vi "Change Configuration.vi"(1 "input cluster":T1 {"MaxLambdaCurrent [A]" format="%.3f"; "LambdaRates [A/min]" format="%.2f"; "MaxNormalCurrent [A]" format="%.3f"; "StabilitySetting [%]" format="%.2f"; "FieldCurrentRatio [T/A]" format="%.6f"; "SwitchWaitTime [s]" format="%.2f"; "SwitchHtrCurrent [mA]" format="%.2f"; "TrainRates [A/min]" format="%.2f"; "NormalRates [A/min]" format="%.2f"; "Breakpts [A]" format="%.3f"}, 3 "VISA session":refnum<visa-resource-name>="GPIB0::22::INSTR") -> (0 "Output cluster":T1 {"MaxLambdaCurrent [A]" format="%.2f"; "LambdaRates [A/min]" format="%.2f"; "MaxNormalCurrent [A]" format="%.2f"; "StabilitySetting [%]" format="%.2f"; "FieldCurrentRatio [T/A]" format="%.2f"; "SwitchWaitTime [s]" format="%.2f"; "SwitchHtrCurrent [mA]" format="%.2f"; "TrainRates [A/min]" format="%.2f"; "NormalRates [A/min]" format="%.2f"; "Breakpts [A]" format="%.2f"})   [LabVIEW 2019]
panel:
  in  "OK Button":bool
  # "Change parameters below then hit OK\nchanges will be written to the PS and \nthe configuration file"
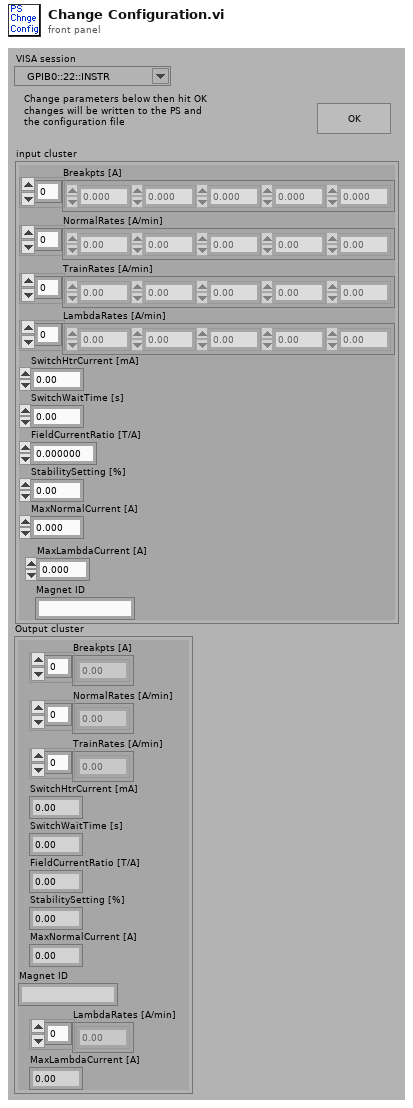
[diagram p1: front panel]
types:
  T1 = cluster{"Breakpts [A]":dbl[], "NormalRates [A/min]":dbl[], "TrainRates [A/min]":dbl[], "SwitchHtrCurrent [mA]":dbl, "SwitchWaitTime [s]":dbl, "FieldCurrentRatio [T/A]":dbl, "StabilitySetting [%]":dbl, "MaxNormalCurrent [A]":dbl, "Magnet ID":string, "LambdaRates [A/min]":dbl[], "MaxLambdaCurrent [A]":dbl}
  T2 = enum16{"Normal", "Train", "Lambda", "Train & Lambda"}
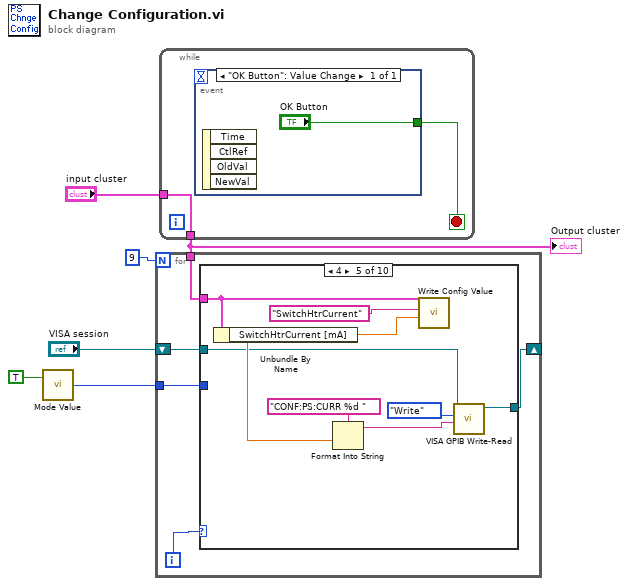
[diagram p0: block diagram]
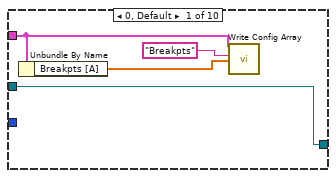
[diagram p2: hidden frame]
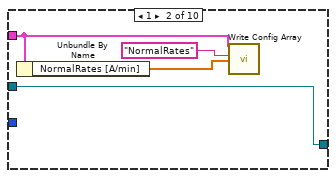
[diagram p3: hidden frame]
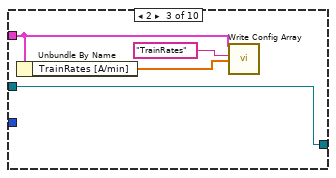
[diagram p4: hidden frame]
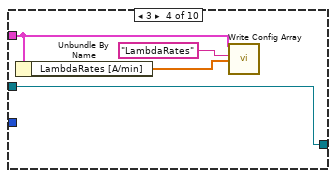
[diagram p5: hidden frame]
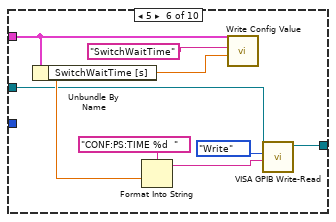
[diagram p6: hidden frame]
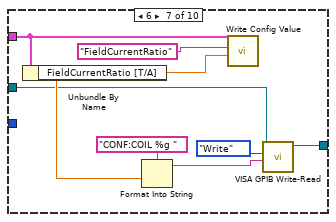
[diagram p7: hidden frame]
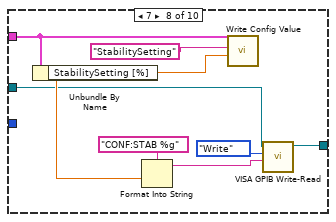
[diagram p8: hidden frame]
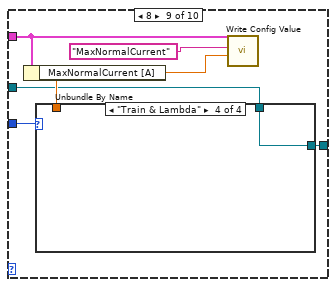
[diagram p9: hidden frame]
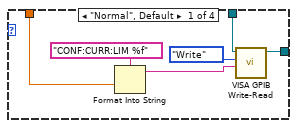
[diagram p10: hidden frame]
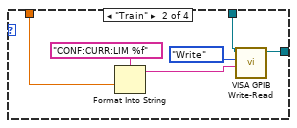
[diagram p11: hidden frame]
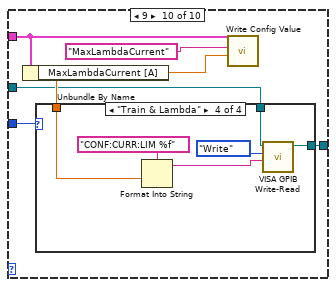
[diagram p13: hidden frame]
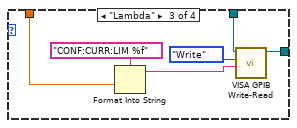
[diagram p16: hidden frame]
diagram:
  n1 = call "Mode Value.vi"("Read/Write this vi"=TRUE) -> ("Mode Out"=w2:T2)  [unwired: 1 in]
  n2 = while {
    tunnel: "input cluster" -> [w7]
    tunnel: [w7] -> w4
    stop <- w8 stop-if-true
    n3 = event shown="[0] \"OK Button\": Value Change" {
      selector: _ -> [_]
      dyn-events: _ -> [_]
      timeout: _ -> [_]
      tunnel: ["OK Button"] -> w8
      event "OK Button": Value Change {
        n4 = event-data() -> ()  [unwired: 1 in, 4 out]
      }
    }
  }
  "Output cluster" <- w4
  n5 = for {
    N: 9 -> [_]
    tunnel: w4 -> [w13]
    tunnel: w2 -> [w12]
    shift-right: [w10] -> _
    shift-left: "VISA session" -> [w11]
    i -> [w14]
    n6 = case shown="4" w14 {
      tunnel: w13 -> [w18 w22 w26 w30 w38 w46 w54 w62 w68 w88]
      tunnel: w12 -> [_ _ _ _ _ _ _ _ w65 w85]
      tunnel: w11 -> [w15 w19 w23 w27 w32 w40 w48 w56 w64 w84]
      tunnel: [w15 w19 w23 w27 w31 w39 w47 w55 w63 w83] -> w10
      frame 0, Default {
        n7 = Unbundle By Name(w18) -> ("Breakpts [A]"=w16:dbl[])
        n8 = call "Write Config Array.vi"("array"=w16, "Key"="Breakpts", "input cluster"=w18) -> ()  [unwired: 1 in, 2 out]
      }
      frame 1 {
        n9 = Unbundle By Name(w22) -> ("NormalRates [A/min]"=w20:dbl[])
        n10 = call "Write Config Array.vi"("array"=w20, "Key"="NormalRates", "input cluster"=w22) -> ()  [unwired: 1 in, 2 out]
      }
      frame 2 {
        n11 = Unbundle By Name(w26) -> ("TrainRates [A/min]"=w24:dbl[])
        n12 = call "Write Config Array.vi"("array"=w24, "Key"="TrainRates", "input cluster"=w26) -> ()  [unwired: 1 in, 2 out]
      }
      frame 3 {
        n13 = Unbundle By Name(w30) -> ("LambdaRates [A/min]"=w28:dbl[])
        n14 = call "Write Config Array.vi"("array"=w28, "Key"="LambdaRates", "input cluster"=w30) -> ()  [unwired: 1 in, 2 out]
      }
      frame 4 {
        n15 = Unbundle By Name(w38) -> ("SwitchHtrCurrent [mA]"=w36:dbl)
        n16 = Format Into String(format string="CONF:PS:CURR %d " ("Command String"), w36) -> (resulting string=w34:string)  [unwired: 2 in, 1 out]
        n17 = call "Write Config Value.vi"("Value"=w36, "Key"="SwitchHtrCurrent", "input cluster"=w38) -> ()  [unwired: 1 in, 2 out]
        n18 = call "VISA GPIB Write-Read.vi"("Command"=w34, "Action"=enum16{"Write", "Read", "Write & Read"}."Write", "VISA resource name"=w32) -> ("dup VISA Session"=w31:refnum<visa-resource-name>)  [unwired: 5 in, 3 out]
      }
      frame 5 {
        n19 = Unbundle By Name(w46) -> ("SwitchWaitTime [s]"=w44:dbl)
        n20 = Format Into String(format string="CONF:PS:TIME %d  " ("Command String"), w44) -> (resulting string=w43:string)  [unwired: 2 in, 1 out]
        n21 = call "Write Config Value.vi"("Value"=w44, "Key"="SwitchWaitTime", "input cluster"=w46) -> ()  [unwired: 1 in, 2 out]
        n22 = call "VISA GPIB Write-Read.vi"("Command"=w43, "Action"=enum16{"Write", "Read", "Write & Read"}."Write", "VISA resource name"=w40) -> ("dup VISA Session"=w39:refnum<visa-resource-name>)  [unwired: 5 in, 3 out]
      }
      frame 6 {
        n23 = Unbundle By Name(w54) -> ("FieldCurrentRatio [T/A]"=w52:dbl)
        n24 = Format Into String(format string="CONF:COIL %g " ("Command String"), w52) -> (resulting string=w50:string)  [unwired: 2 in, 1 out]
        n25 = call "Write Config Value.vi"("Value"=w52, "Key"="FieldCurrentRatio", "input cluster"=w54) -> ()  [unwired: 1 in, 2 out]
        n26 = call "VISA GPIB Write-Read.vi"("Command"=w50, "Action"=enum16{"Write", "Read", "Write & Read"}."Write", "VISA resource name"=w48) -> ("dup VISA Session"=w47:refnum<visa-resource-name>)  [unwired: 5 in, 3 out]
      }
      frame 7 {
        n27 = Unbundle By Name(w62) -> ("StabilitySetting [%]"=w60:dbl)
        n28 = Format Into String(format string="CONF:STAB %g" ("Command String"), w60) -> (resulting string=w58:string)  [unwired: 2 in, 1 out]
        n29 = call "Write Config Value.vi"("Value"=w60, "Key"="StabilitySetting", "input cluster"=w62) -> ()  [unwired: 1 in, 2 out]
        n30 = call "VISA GPIB Write-Read.vi"("Command"=w58, "Action"=enum16{"Write", "Read", "Write & Read"}."Write", "VISA resource name"=w56) -> ("dup VISA Session"=w55:refnum<visa-resource-name>)  [unwired: 5 in, 3 out]
      }
      frame 8 {
        n31 = Unbundle By Name(w68) -> ("MaxNormalCurrent [A]"=w66:dbl)
        n32 = case shown="\"Train & Lambda\"" w65 {
          tunnel: w66 -> [w74 w80 _ _]
          tunnel: w64 -> [w70 w76 w81 w82]
          tunnel: [w69 w75 w81 w82] -> w63
          frame "Normal", Default {
            n33 = Format Into String(format string="CONF:CURR:LIM %f" ("Command String"), w74) -> (resulting string=w72:string)  [unwired: 2 in, 1 out]
            n34 = call "VISA GPIB Write-Read.vi"("Command"=w72, "Action"=enum16{"Write", "Read", "Write & Read"}."Write", "VISA resource name"=w70) -> ("dup VISA Session"=w69:refnum<visa-resource-name>)  [unwired: 5 in, 3 out]
          }
          frame "Train" {
            n35 = Format Into String(format string="CONF:CURR:LIM %f" ("Command String"), w80) -> (resulting string=w78:string)  [unwired: 2 in, 1 out]
            n36 = call "VISA GPIB Write-Read.vi"("Command"=w78, "Action"=enum16{"Write", "Read", "Write & Read"}."Write", "VISA resource name"=w76) -> ("dup VISA Session"=w75:refnum<visa-resource-name>)  [unwired: 5 in, 3 out]
          }
          frame "Lambda" {
          }
          frame "Train & Lambda" {
          }
        }
        n37 = call "Write Config Value.vi"("Value"=w66, "Key"="MaxNormalCurrent", "input cluster"=w68) -> ()  [unwired: 1 in, 2 out]
      }
      frame 9 {
        n38 = Unbundle By Name(w88) -> ("MaxLambdaCurrent [A]"=w86:dbl)
        n39 = case shown="\"Train & Lambda\"" w85 {
          tunnel: w86 -> [_ _ w96 w102]
          tunnel: w84 -> [w89 w90 w92 w98]
          tunnel: [w89 w90 w91 w97] -> w83
          frame "Normal", Default {
          }
          frame "Train" {
          }
          frame "Lambda" {
            n40 = Format Into String(format string="CONF:CURR:LIM %f" ("Command String"), w96) -> (resulting string=w94:string)  [unwired: 2 in, 1 out]
            n41 = call "VISA GPIB Write-Read.vi"("Command"=w94, "Action"=enum16{"Write", "Read", "Write & Read"}."Write", "VISA resource name"=w92) -> ("dup VISA Session"=w91:refnum<visa-resource-name>)  [unwired: 5 in, 3 out]
          }
          frame "Train & Lambda" {
            n42 = Format Into String(format string="CONF:CURR:LIM %f" ("Command String"), w102) -> (resulting string=w100:string)  [unwired: 2 in, 1 out]
            n43 = call "VISA GPIB Write-Read.vi"("Command"=w100, "Action"=enum16{"Write", "Read", "Write & Read"}."Write", "VISA resource name"=w98) -> ("dup VISA Session"=w97:refnum<visa-resource-name>)  [unwired: 5 in, 3 out]
          }
        }
        n44 = call "Write Config Value.vi"("Value"=w86, "Key"="MaxLambdaCurrent", "input cluster"=w88) -> ()  [unwired: 1 in, 2 out]
      }
    }
  }
